vi "Read_pathWeaver_JSON_File.vi"() -> ()   [LabVIEW 2019]
uses:
  <vilib>/Rock Robotics/WPI/ThirdParty/JAS_Junk/TrajLib/TRAJECTORY.ctl
  <vilib>/Rock Robotics/WPI/ThirdParty/JAS_Junk/TrajLib/TRAJ_STATE.ctl
  <vilib>/Rock Robotics/WPI/ThirdParty/JAS_Junk/TrajLib/POSE2D.ctl
  <vilib>/Rock Robotics/WPI/ThirdParty/JAS_Junk/TrajLib/TRANSLATION2D.ctl
  <vilib>/Rock Robotics/WPI/ThirdParty/JAS_Junk/TrajLib/ROTATION2D.ctl
  <vilib>/Rock Robotics/WPI/ThirdParty/JAS_Junk/TrajLib/Trajectory_Library.lvlib
panel:
  out "TotalTImeSecs":dbl
  out "error out":errorcluster
  out "outTRAJECTORY":T1 {"TotalTImeSecs" format="%20.3f"}
  in  "Tab Control 2":enum32{"Read JSON FILE"}(tab)
  in  "CreateCmdList 2":bool
  in  "json file name":path
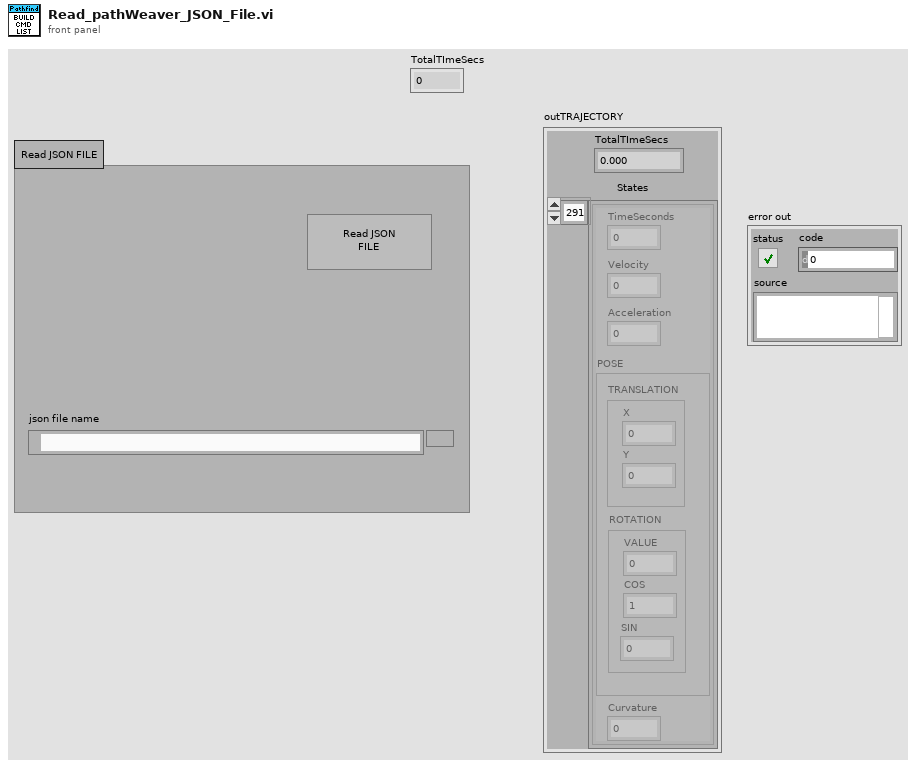
[diagram p1: front panel]
types:
  T1 = typedef "Trajectory_Library.lvlib/TRAJECTORY.ctl" = cluster{"TotalTImeSecs":dbl, "States":T2[]}
  T2 = typedef "Trajectory_Library.lvlib/TRAJ_STATE.ctl" = cluster{"TimeSeconds":dbl, "Velocity":dbl, "Acceleration":dbl, "POSE":T3, "Curvature":dbl}
  T3 = typedef "Trajectory_Library.lvlib/POSE2D.ctl" = cluster{"TRANSLATION":T4, "ROTATION":T5}
  T4 = typedef "Trajectory_Library.lvlib/TRANSLATION2D.ctl" = cluster{"X":dbl, "Y":dbl}
  T5 = typedef "Trajectory_Library.lvlib/ROTATION2D.ctl" = cluster{"VALUE":dbl, "COS":dbl, "SIN":dbl}
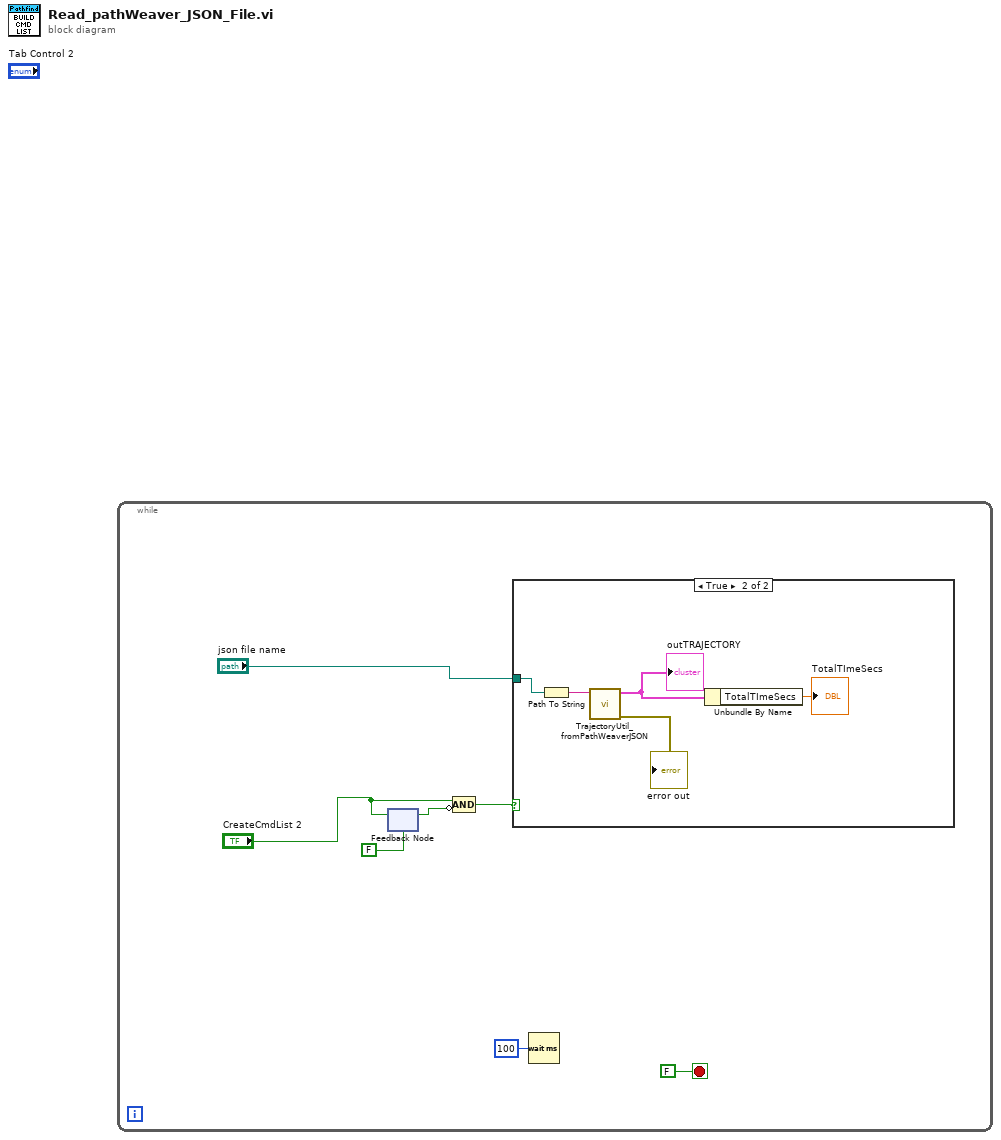
[diagram p0: block diagram]
diagram:
  n1 = while {
    stop <- FALSE stop-if-true
    n2 = feedback-in #1("CreateCmdList 2") -> ()
    n3 = feedback #1(FALSE) -> (w4:bool)
    n4 = Compound Arithmetic op=AND("CreateCmdList 2", invert w4) -> (w1:bool)
    n5 = case shown="True" w1 {
      tunnel: "json file name" -> [_ w11]
      frame False {
      }
      frame True {
        n6 = Path To String(path=w11) -> (string=w12:string)
        n7 = call <vilib>:"TrajectoryUtil_fromPathWeaverJSON.vi"("FileName"=w12) -> ("error out"=→"error out":errorcluster, "outTRAJECTORY"=w9:T1)  [unwired: 9 in]
        "outTRAJECTORY" <- w9
        n8 = Unbundle By Name(w9) -> ("TotalTImeSecs"=→"TotalTImeSecs":dbl)
      }
    }
    n9 = Wait (ms)(milliseconds to wait=u32 100) -> ()  [unwired: 1 out]
  }
